vi "Send ADC.vi"(8 "error in (no error)":errorcluster, 9 "VISA resource name":refnum<visa-resource-name>, 10 "Channel ADC":u16, 11 "Simulada in":refnum<class "Simulada.lvclass">) -> (0 "error out":errorcluster, 1 "ADC Value":dbl, 2 "VISA resource name 2":refnum<visa-resource-name>, 3 "Simulada out":refnum<class "Simulada.lvclass">)   [LabVIEW 2020, in "Simulada.lvclass"]
uses:
  Simulada.lvclass
  Abstract/Serial Device/Serial Device.lvclass
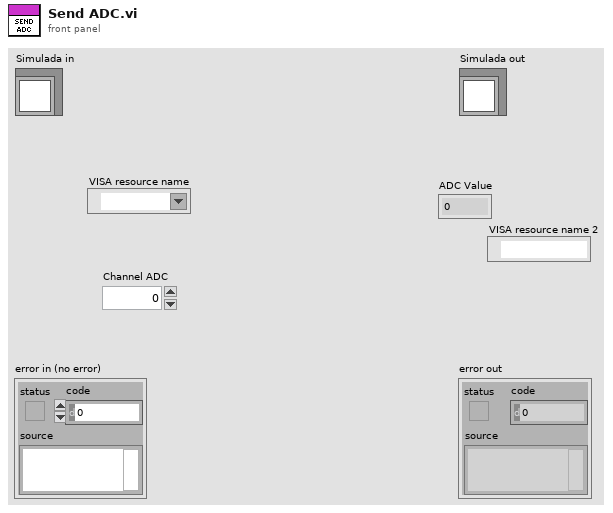
[diagram p1: front panel]
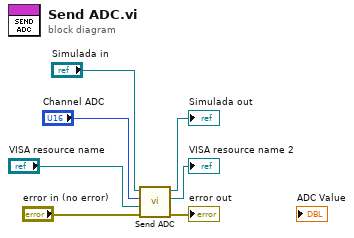
[diagram p0: block diagram]
diagram:
  n1 = call-parent "Send ADC.vi"("error in (no error)"="error in (no error)", "VISA resource name"="VISA resource name", "Channel ADC"="Channel ADC", "Serial Device in"="Simulada in") -> ("error out"=→"error out":errorcluster, "VISA resource name 2"=→"VISA resource name 2":refnum<visa-resource-name>, "Serial Device out"=→"Simulada out":refnum<class "Simulada.lvclass">)  [unwired: 4 in, 1 out]
